vi "Build String Array.vi"(7 "Initialize":bool, 10 "string":string) -> (2 "Array":string[](array[string]))   [LabVIEW 2016]
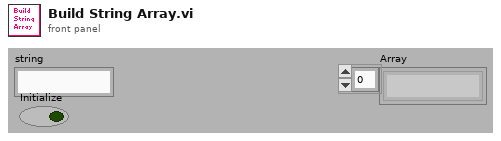
[diagram p1: front panel]
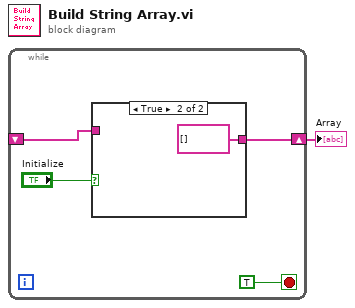
[diagram p0: block diagram]
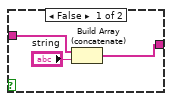
[diagram p2: hidden frame]
diagram:
  n1 = while {
    shift-right: [w4] -> w1
    shift-left: _ -> [w5]
    stop <- TRUE stop-if-true
    n2 = case shown="True" "Initialize" {
      tunnel: w5 -> [w8 _]
      tunnel: [w7 string[] []] -> w4
      frame False {
        n3 = Build Array (concatenate)(w8, "string") -> (w7:string[])
      }
      frame True {
      }
    }
  }
  "Array" <- w1
